vi "FreqDivider.vi"() -> ()   [LabVIEW 2020]
uses:
  <vilib>/DAQmx/create/channels.llb/DAQmx Create Channel (CO-Pulse Generation-Frequency).vi
  <vilib>/DAQmx/configure/timing.llb/DAQmx Timing (Implicit).vi
  <vilib>/DAQmx/create/channels.llb/DAQmx Create Channel (CO-Pulse Generation-Ticks).vi
  <resource>/objmgr/daqmx.rc
panel:
  in  "Output Pulse":tag
  in  "Input Pulse":tag
  in  "counter 2":tag
  out "Output Frequency":dbl
  in  "counter":tag
  in  "stop":bool
  in  "Input Frequency":dbl=1.0 min=1.0 max=25000000.0 step=1000.0
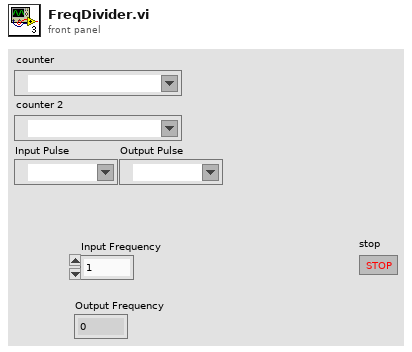
[diagram p1: front panel]
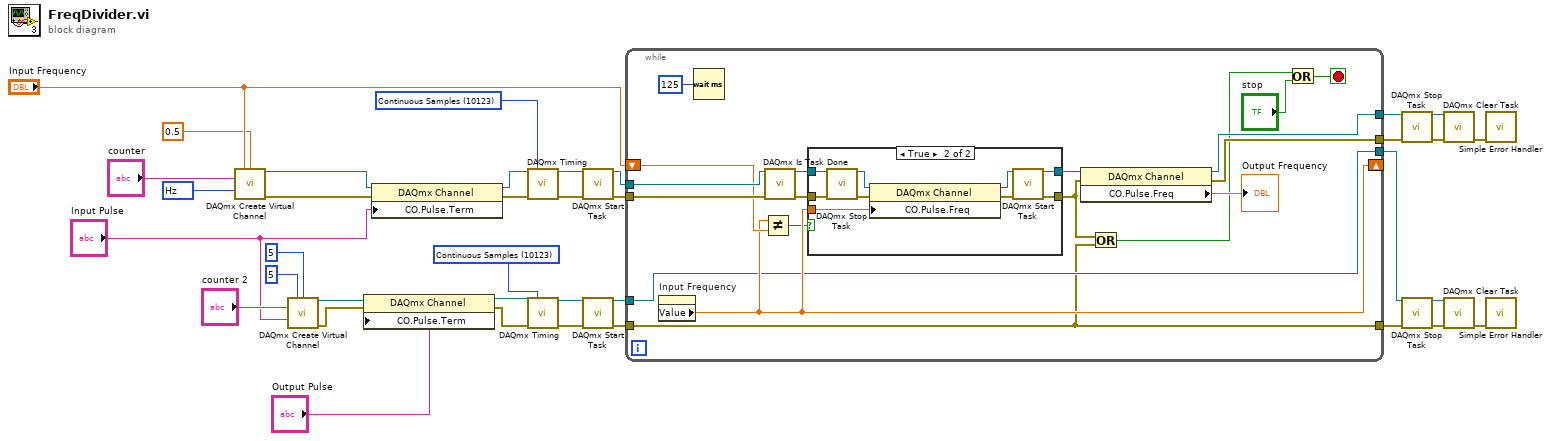
[diagram p0: block diagram]
diagram:
  w11 = 10123 items=["Finite Samples"=10178, "Continuous Samples"=10123, "Hardware Timed Single Point"=12522] ("sample mode")
  w36 = 10123 items=["Finite Samples"=10178, "Continuous Samples"=10123, "Hardware Timed Single Point"=12522] ("sample mode")
  w37 = 10373 items=["Hz"=10373] ("units")
  n1 = call-poly <vilib>:"DAQmx Create Virtual Channel.vi"("frequency"="Input Frequency", "duty cycle"=0.5, "counter"="counter", "units"=w37) -> ("task out"=w22:refnum<k21>, "error out"=w21:errorcluster)  [unwired: 10 in]
  n2 = call-poly <vilib>:"DAQmx Create Virtual Channel.vi"("high ticks"=u32 5, "low ticks"=u32 5, "counter"="counter 2", "source of ticks"="Input Pulse") -> ("task out"=w5:refnum<k21>, "error out"=w4:errorcluster)  [unwired: 10 in]
  n3 = property class="DAQmx Channel"(reference=w5, error in=w4, "CO.Pulse.Term"="Output Pulse") -> (reference out=w3:refnum<k21>, error out=w2:errorcluster)
  n4 = property class="DAQmx Channel"(reference=w22, error in=w21, "CO.Pulse.Term"="Input Pulse") -> (reference out=w20:refnum<k21>, error out=w19:errorcluster)
  n5 = call-poly <vilib>:"DAQmx Timing.vi"("task/channels in"=w20, "sample mode"=w36, "error in"=w19) -> ("task out"=w35:refnum<k21>, "error out"=w34:errorcluster)  [unwired: 11 in]
  n6 = call-poly <vilib>:"DAQmx Timing.vi"("task/channels in"=w3, "sample mode"=w11, "error in"=w2) -> ("task out"=w15:refnum<k21>, "error out"=w14:errorcluster)  [unwired: 11 in]
  n7 = call <vilib>:"DAQmx Start Task.vi"("task/channels in"=w35, "error in"=w34) -> ("task out"=w33:refnum<k21>, "error out"=w32:errorcluster)  [unwired: 12 in]
  n8 = call <vilib>:"DAQmx Start Task.vi"("task/channels in"=w15, "error in"=w14) -> ("task out"=w13:refnum<k21>, "error out"=w12:errorcluster)  [unwired: 12 in]
  n9 = while {
    tunnel: w33 -> [w55]
    tunnel: w32 -> [w54]
    shift-right: [w45] -> _
    shift-left: "Input Frequency" -> [w49]
    tunnel: [w44] -> w26
    tunnel: [w43] -> w25
    tunnel: w13 -> [w41]
    tunnel: w12 -> [w39]
    tunnel: [w41] -> w7
    tunnel: [w39] -> w6
    stop <- w51 stop-if-true
    n10 = property on="Input Frequency" class="DigNum (strict)"() -> ("Value"=w45:dbl)  [unwired: 2 in, 2 out]
    n11 = Wait (ms)(milliseconds to wait=u32 125) -> ()  [unwired: 1 out]
    n12 = Not Equal?(x=w45, y=w49) -> (x != y?=w42:bool)
    n13 = call <vilib>:"DAQmx Is Task Done.vi"("task/channels in"=w55, "error in"=w54) -> ("task out"=w53:refnum<k21>, "error out"=w52:errorcluster)  [unwired: 11 in, 1 out]
    n14 = case shown="True" w42 {
      tunnel: w53 -> [w57 w65]
      tunnel: w52 -> [w56 w64]
      tunnel: w45 -> [_ w66]
      tunnel: [w57 w61] -> w47
      tunnel: [w56 w60] -> w40
      frame False {
      }
      frame True {
        n15 = call <vilib>:"DAQmx Stop Task.vi"("task/channels in"=w65, "error in"=w64) -> ("task out"=w63:refnum<k21>, "error out"=w62:errorcluster)  [unwired: 12 in]
        n16 = property class="DAQmx Channel"(reference=w63, error in=w62, "CO.Pulse.Freq"=w66) -> (reference out=w58:refnum<k21>, error out=w59:errorcluster)
        n17 = call <vilib>:"DAQmx Start Task.vi"("task/channels in"=w58, "error in"=w59) -> ("task out"=w61:refnum<k21>, "error out"=w60:errorcluster)  [unwired: 12 in]
      }
    }
    n18 = property class="DAQmx Channel"(reference=w47, error in=w40) -> (reference out=w44:refnum<k21>, error out=w43:errorcluster, "CO.Pulse.Freq"=→"Output Frequency":dbl)
    n19 = Or(x=w40, y=w39) -> (x .or. y?=w38:bool)
    n20 = Or(x=w38, y="stop") -> (x .or. y?=w51:bool)
  }
  n21 = call <vilib>:"DAQmx Stop Task.vi"("task/channels in"=w26, "error in"=w25) -> ("task out"=w30:refnum<k21>, "error out"=w29:errorcluster)  [unwired: 12 in]
  n22 = call <vilib>:"DAQmx Stop Task.vi"("task/channels in"=w7, "error in"=w6) -> ("task out"=w10:refnum<k21>, "error out"=w9:errorcluster)  [unwired: 12 in]
  n23 = call <vilib>:"DAQmx Clear Task.vi"("task in"=w30, "error in"=w29) -> ("error out"=w28:errorcluster)  [unwired: 13 in]
  n24 = call <vilib>:"DAQmx Clear Task.vi"("task in"=w10, "error in"=w9) -> ("error out"=w8:errorcluster)  [unwired: 13 in]
  n25 = call <vilib>:"Simple Error Handler.vi"("error in (no error)"=w28) -> ()  [unwired: 4 in, 5 out]
  n26 = call <vilib>:"Simple Error Handler.vi"("error in (no error)"=w8) -> ()  [unwired: 4 in, 5 out]
